vi "RVC 8-link serial robot.vi"() -> ()   [LabVIEW 2013]
uses:
  <vilib>/Analysis/Matrix/Datatypes/RealMatrix.ctl
  <vilib>/robotics/Kinematics/Analytical/Initialize Generic Serial Arm.vi
  <vilib>/robotics/Kinematics/Robot/Forward Kinematics (Point).vi
  <vilib>/picture/3D Picture Control/Object/Add Object (no reference).vi
  <vilib>/robotics/Kinematics/Analytical/NI_Robotics_AnalyticKinematics.lvlib
  <vilib>/robotics/Kinematics/Plotting/NI_Robotics_3DKinematics.lvlib
  <vilib>/picture/3D Picture Control/NI_3D Picture Control.lvlib
  <vilib>/robotics/Kinematics/NI_Kinematics.lvlib
  <vilib>/robotics/Kinematics/Robot/NI_Robotics_Serial Robot Arm.lvclass
  <vilib>/robotics/Kinematics/Link/Joint Type.ctl
  <vilib>/robotics/Kinematics/Link/NI_Robotics_Link.lvclass
  <vilib>/Analysis/Matrix/NI_Matrix.lvlib
panel:
  out "forward kinematics":T1
  out "3D Picture":refnum<vi>(3d-picture)
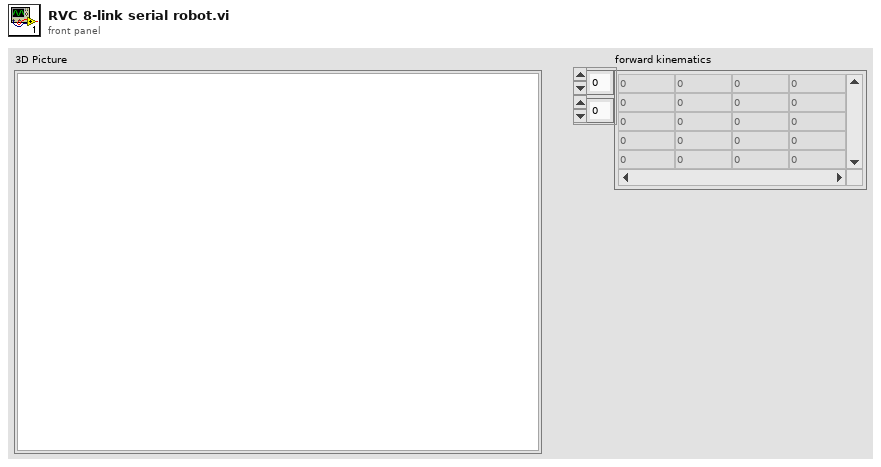
[diagram p1: front panel]
types:
  T1 = typedef "NI_Matrix.lvlib/RealMatrix.ctl" = dbl[][]
  T2 = typedef "NI_Robotics_Link.lvclass/Joint Type.ctl" = enum16{"Revolute", "Prismatic"}
  T3 = cluster{"Twist Angle":dbl, "Length":dbl, "Rotation Angle":dbl, "Offset Distance":dbl, "Joint Type":T2, "Joint Coordinate Offset":dbl}[]
  T4 = typedef "DH Kinematic Parameters.ctl" = cluster{"twist angle":dbl, "length":dbl, "rotation angle":dbl, "offset distance":dbl, "joint type":T2, "joint coordinate offset":dbl}
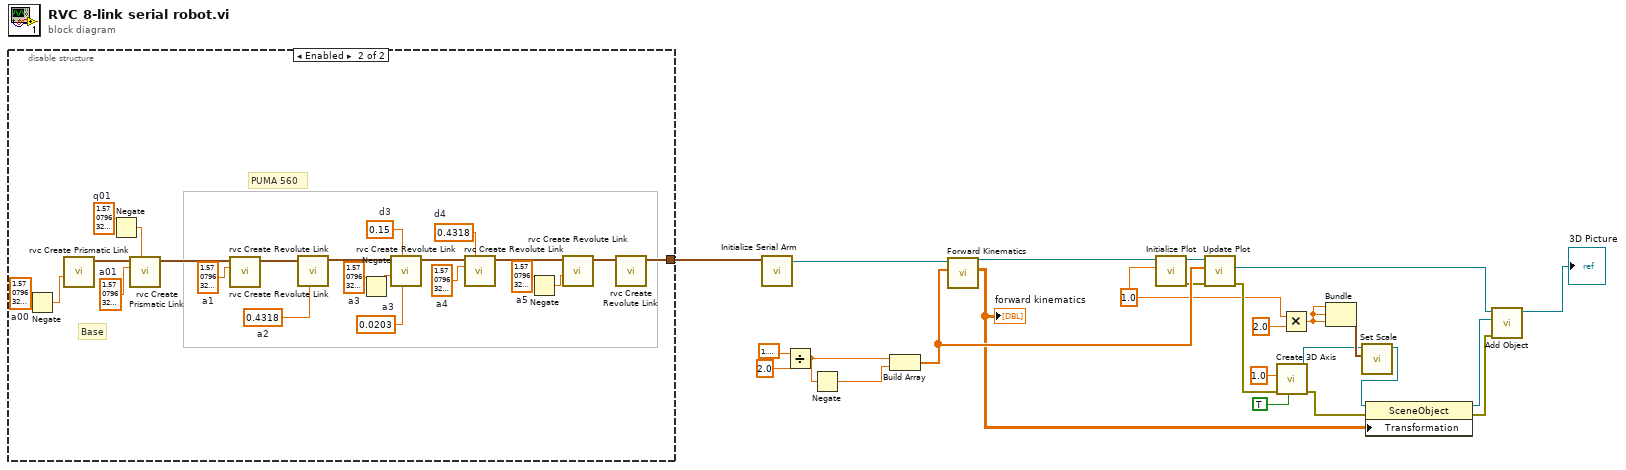
[diagram p0: block diagram]
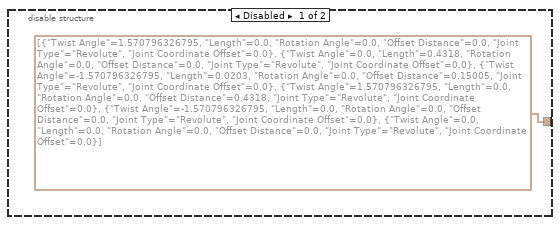
[diagram p2: hidden frame]
diagram:
  w6 = 1.0 ("scale (1)")
  n1 = disable-structure shown="Enabled" {
    disable-tunnel: [T3 [{"Twist Angle"=1.570796326795, "Length"=0.0, "Rotation Angle"=0.0, "Offset Distance"=0.0, "Joint Type"=enum."Revolute", "Joint Coordinate Offset"=0.0}, {"Twist Angle"=0.0, "Length"=0.4318, "Rotation Angle"=0.0, "Offset Distance"=0.0, "Joint Type"=enum."Revolute", "Joint Coordinate Offset"=0.0}, {"Twist Angle"=-1.570796326795, "Length"=0.0203, "Rotation Angle"=0.0, "Offset Distance"=0.15005, "Joint Type"=enum."Revolute", "Joint Coordinate Offset"=0.0}, {"Twist Angle"=1.570796326795, "Length"=0.0, "Rotation Angle"=0.0, "Offset Distance"=0.4318, "Joint Type"=enum."Revolute", "Joint Coordinate Offset"=0.0}, {"Twist Angle"=-1.570796326795, "Length"=0.0, "Rotation Angle"=0.0, "Offset Distance"=0.0, "Joint Type"=enum."Revolute", "Joint Coordinate Offset"=0.0}, {"Twist Angle"=0.0, "Length"=0.0, "Rotation Angle"=0.0, "Offset Distance"=0.0, "Joint Type"=enum."Revolute", "Joint Coordinate Offset"=0.0}] w48] -> w25
    frame Disabled {
    }
    frame Enabled {
      w28 = 1.5707963267948966  # q01
      w29 = 1.5707963267948966  # a01
      w31 = 1.5707963267948966  # a00
      w35 = 1.5707963267948966  # a5
      w36 = 0.4318  # d4
      w37 = 1.5707963267948966  # a4
      w39 = 1.5707963267948966  # a3
      w40 = 0.15  # d3
      w41 = 0.0203  # a3
      w45 = 0.4318  # a2
      w47 = 1.5707963267948966  # a1
      # "Base"
      # "PUMA 560"
      n2 = Negate(x=w31) -> (-x=w30:dbl)
      n3 = call "rvc Create Prismatic Link.vi"("twist angle (alpha)"=w30) -> ("Array"=w33:T4[])  [unwired: 10 in]
      n4 = Negate(x=w28) -> (-x=w27:dbl)
      n5 = call "rvc Create Prismatic Link.vi"("rotation angle (theta)"=w27, "twist angle (alpha)"=w29, "Array 2"=w33) -> ("Array"=w32:T4[])  [unwired: 8 in]
      n6 = call "rvc Create Revolute Link.vi"("twist angle (alpha)"=w47, "Array 2"=w32) -> ("Array"=w46:T4[])  [unwired: 9 in]
      n7 = call "rvc Create Revolute Link.vi"("length (a)"=w45, "Array 2"=w46) -> ("Array"=w44:T4[])  [unwired: 9 in]
      n8 = Negate(x=w39) -> (-x=w38:dbl)
      n9 = call "rvc Create Revolute Link.vi"("length (a)"=w41, "offset distance (d)"=w40, "twist angle (alpha)"=w38, "Array 2"=w44) -> ("Array"=w43:T4[])  [unwired: 7 in]
      n10 = call "rvc Create Revolute Link.vi"("offset distance (d)"=w36, "twist angle (alpha)"=w37, "Array 2"=w43) -> ("Array"=w42:T4[])  [unwired: 8 in]
      n11 = Negate(x=w35) -> (-x=w34:dbl)
      n12 = call "rvc Create Revolute Link.vi"("twist angle (alpha)"=w34, "Array 2"=w42) -> ("Array"=w49:T4[])  [unwired: 9 in]
      n13 = call "rvc Create Revolute Link.vi"("Array 2"=w49) -> ("Array"=w48:T4[])  [unwired: 10 in]
    }
  }
  n14 = call-poly <vilib>:"Initialize Serial Arm.vi"("kinematic parameters"=w25) -> ("serial arm out"=w24:refnum<class "NI_Robotics_Serial Robot Arm.lvclass">)  [unwired: 9 in, 1 out]
  n15 = Divide(x=1.5707963267948966, y=2.0) -> (x/y=w13:dbl)
  n16 = Negate(x=w13) -> (-x=w12:dbl)
  n17 = Build Array(w13, w12) -> (w19:dbl[])
  n18 = call-poly <vilib>:"Forward Kinematics.vi"("joint positions"=w19, "serial arm in"=w24) -> ("end effector transform"=w17:T1, "serial arm out"=w23:refnum<class "NI_Robotics_Serial Robot Arm.lvclass">)  [unwired: 7 in, 1 out]
  "forward kinematics" <- w17
  n19 = call <vilib>:"Initialize Plot.vi"("scale (1)"=w6, "serial arm in"=w23) -> ("error out"=w11:errorcluster, "serial arm out"=w22:refnum<class "NI_Robotics_Serial Robot Arm.lvclass">)  [unwired: 8 in]
  n20 = call <vilib>:"Update Plot.vi"("error in (no error)"=w11, "joint positions"=w19, "serial arm in"=w22) -> ("error out"=w10:errorcluster, "serial arm scene"=w18:refnum<vi>)  [unwired: 6 in, 1 out]
  n21 = call <vilib>:"Create 3D Axis.vi"("Axis label?"=TRUE, "error in (no error)"=w10, "Length"=sgl 1.0) -> ("error out"=w9:errorcluster, "New Object Refnum"=w3:refnum<vi>)  [unwired: 7 in]
  n22 = Multiply(x=w6, y=2.0) -> (x*y=w5:dbl)
  n23 = Bundle(w5, w5, w5) -> (w4:cluster{dbl, dbl, dbl})  [unwired: 1 in]
  n24 = call <vilib>:"Set Scale.vi"("Scale"=w4, "Scene Object"=w3) -> ("Scaled Object"=w2:refnum<vi>)  [unwired: 8 in, 1 out]
  n25 = property class="SceneObject"(reference=w2, error in=w9, "Transformation"=w17) -> (reference out=w1:refnum<vi>, error out=w8:errorcluster)
  n26 = call-poly <vilib>:"Add Object.vi"("error in (no error)"=w8, "New Object In"=w1, "Scene Object In"=w18) -> ("Scene Object Out"=→"3D Picture":refnum<vi>)  [unwired: 7 in, 1 out]
